vi "Execute Time Elapsed.vi"(8 "error in (no error)":errorcluster, 10 "Time Elapsed":dbl format="%#_13g", 11 "Chef Actor in":refnum<class "Chef Actor.lvclass">) -> (0 "error out":errorcluster, 3 "Chef Actor out":refnum<class "Chef Actor.lvclass">)   [LabVIEW 2024, in "Chef Actor.lvlib" / "Chef Actor.lvclass"]
uses:
  Chef Actor.lvclass
  Chef Actor.lvclass/Chef Actor.ctl
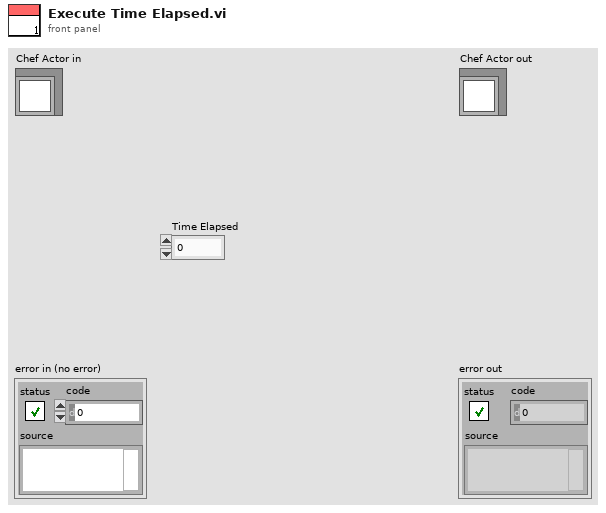
[diagram p1: front panel]
types:
  T1 = typedef "Step.ctl" = cluster{"Fire":dbl, "Duration":dbl}
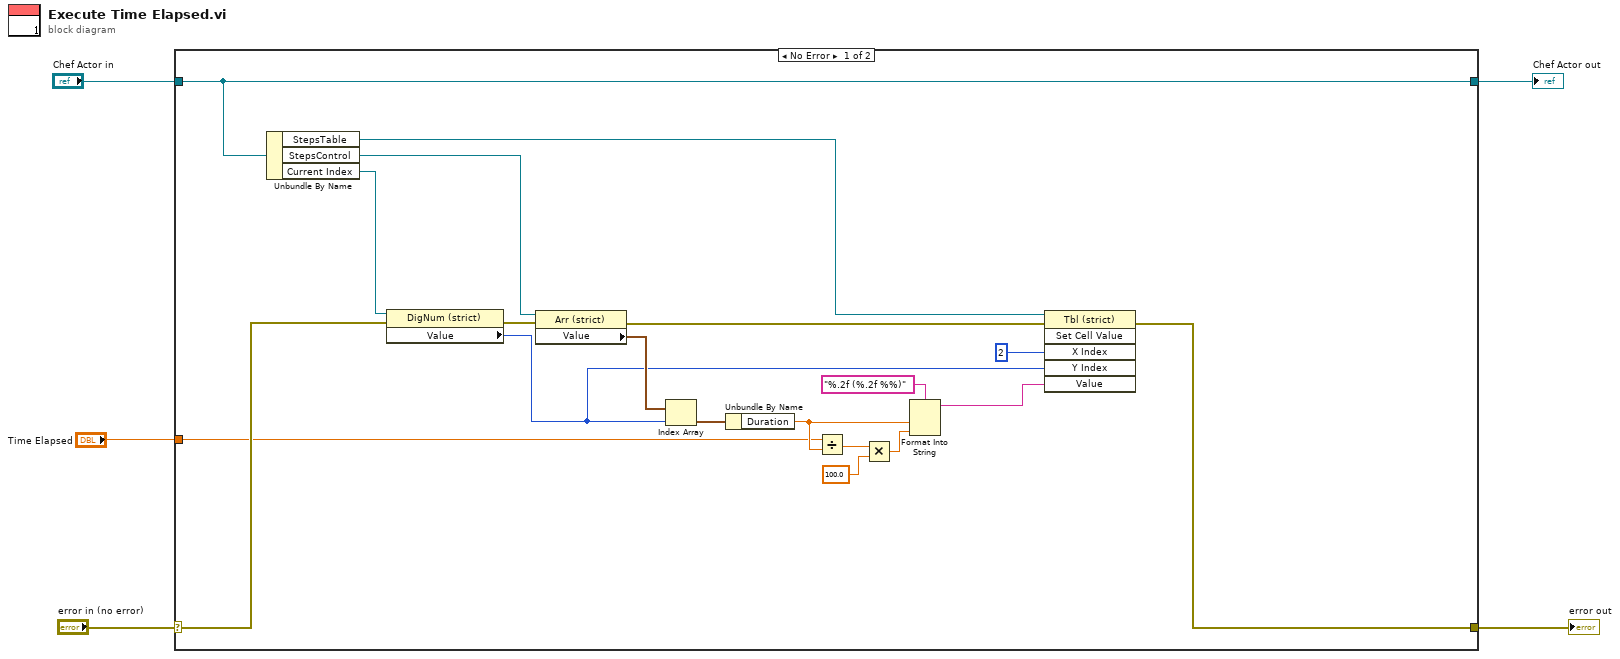
[diagram p0: block diagram]
diagram:
  n1 = case shown="No Error" "error in (no error)" {
    selector: "error in (no error)" -> [w22 w26]
    tunnel: [w6 w26] -> w4
    tunnel: [w24 w25] -> w2
    tunnel: "Chef Actor in" -> [w24 w25]
    tunnel: "Time Elapsed" -> [w10 _]
    frame No Error {
      n2 = Unbundle By Name(w24) -> ("StepsTable"=w7:refnum<vi>, "StepsControl"=w13:refnum<vi>, "Current Index"=w23:refnum<vi>)
      n3 = property class="DigNum (strict)"(reference=w23, error in=w22) -> (error out=w12:errorcluster, "Value"=w8:i32)  [unwired: 1 out]
      n4 = property class="Arr (strict)"(reference=w13, error in=w12) -> (error out=w9:errorcluster, "Value"=w11:T1[])  [unwired: 1 out]
      n5 = Index Array(array=w11, index=w8) -> (element=w21:T1)
      n6 = Unbundle By Name(w21) -> ("Duration"=w16:dbl)
      n7 = Divide(x=w10, y=w16) -> (x/y=w20:dbl)
      n8 = Multiply(x=w20, y=100.0) -> (x*y=w17:dbl)
      n9 = Format Into String(format string="%.2f (%.2f %%)", w16, w17) -> (resulting string=w15:string)  [unwired: 2 in, 1 out]
      n10 = invoke on="Invoke Node" class="Tbl (strict)" method="Set Cell Value"(reference=w7, error in=w9, "X Index"=2 ("index (col)"), "Y Index"=w8, "Value"=w15) -> (error out=w6:errorcluster)  [unwired: 1 in, 5 out]
    }
    frame Error {
    }
  }
  "error out" <- w4
  "Chef Actor out" <- w2
